vi "errorCodesAndMessages.vi"() -> (1 "errorCodes":i32[](array[numeric]), 2 "errorMessages":string[](array[string]))   [LabVIEW 2013]
uses:
  Ctrls/EnumErrors.ctl
panel:
  in  "EnumErreurs":T1
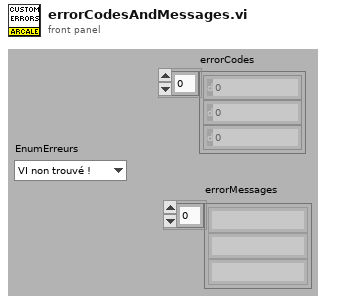
[diagram p1: front panel]
types:
  T1 = typedef "EnumErrors.ctl" = enum16{"VI non trouvé !", "Clé non trouvée", "Timeout", "Le VI tourne déjà", "Erreur de séparateur décimal", "Référence non trouvée"}
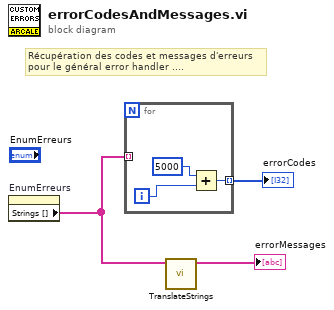
[diagram p0: block diagram]
diagram:
  # "Récupération des codes et messages d'erreurs\npour le général error handler ...."
  n1 = property on="EnumErreurs" class="Enum (strict)"() -> ("Strings []"=w2:string[])  [unwired: 2 in, 2 out]
  n2 = for {
    tunnel: w2 -> [_] mode=indexing
    tunnel: [w4] -> w3 mode=indexing
    i -> [w5]
    n3 = Add(x=5000, y=w5) -> (x+y=w4:i32)
  }
  "errorCodes" <- w3
  n4 = call "TranslateStrings.vi"("String Array"=w2) -> ("Translated string array"=→"errorMessages":string[])  [unwired: 9 in, 1 out]
